vi "Z_Alignment_v12 (SubVI).vi"(4 "System no.":i32, 5 "Z range":dbl, 6 "Intensity Graph":dbl[][](array[numeric]), 7 "Z Mesh":dbl, 8 "error in (no error)":errorcluster, 9 "Z":dbl, 10 "Y":dbl, 11 "X":dbl) -> (0 "error out":errorcluster, 1 "Zout":dbl)   [LabVIEW 2023]
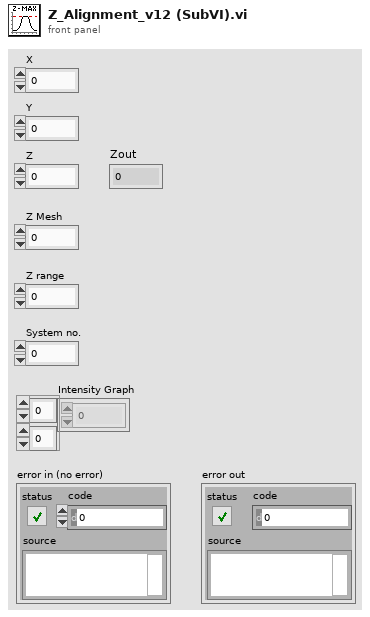
[diagram p1: front panel]
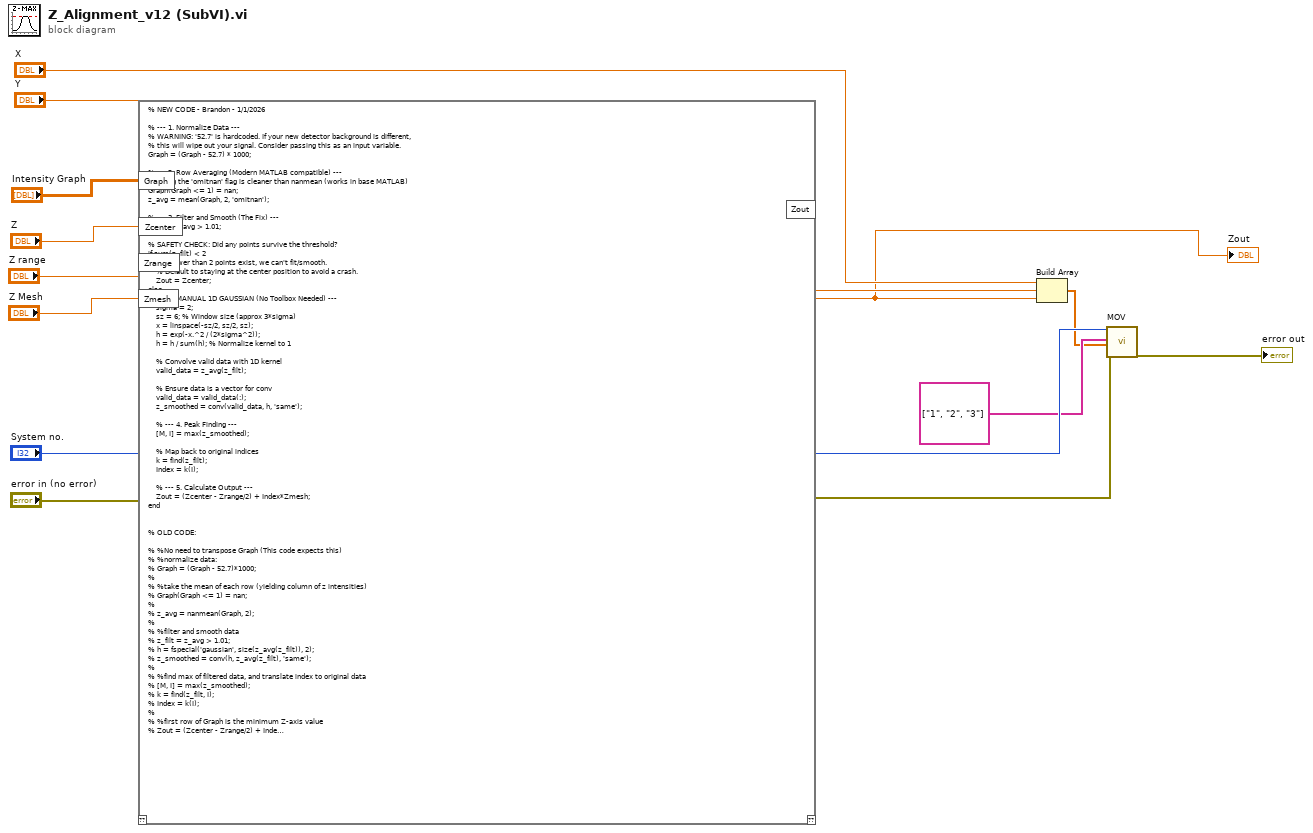
[diagram p0: block diagram]
diagram:
  n1 = script code="% NEW CODE - Brandon - 1/1/2026\n\n% --- 1. Normalize Data ---\n% WARNING: '52.7' is hardcoded. If your new detector background is different,\n% this will wipe out your signal. Consider passing this as an input variable.\nGraph = (Graph - 52.7) * 1000;\n\n% --- 2. Row Averaging (Modern MATLAB compatible) ---\n% Using the 'omitnan' flag is cleaner than nanmean (works in base MATLAB)\nGraph(Graph <= 1) = nan;\nz_avg = mean(Graph, 2, 'omitnan');\n\n% --- 3. Filter and Smooth (The Fix) ---\nz_filt = z_avg > 1.01;\n\n% SAFETY CHECK: Did any points survive the threshold?\nif sum(z_filt) < 2\n    % If fewer than 2 points exist, we can't fit/smooth. \n    % Default to staying at the center position to avoid a crash.\n    Zout = Zcenter; \nelse\n    % --- MANUAL 1D GAUSSIAN (No Toolbox Needed) ---\n    sigma = 2; \n    sz = 6; % Window size (approx 3*sigma)\n    x = linspace(-sz/2, sz/2, sz);\n    h = exp(-x.^2 / (2*sigma^2));\n    h = h / sum(h); % Normalize kernel to 1\n\n    % Convolve valid data with 1D kernel\n    valid_data = z_avg(z_filt);\n    \n    % Ensure data is a vector for conv\n    valid_data = valid_data(:); \n    z_smoothed = conv(valid_data, h, 'same');\n\n    % --- 4. Peak Finding ---\n    [M, I] = max(z_smoothed);\n    \n    % Map back to original indices\n    k = find(z_filt);\n    Index = k(I);\n\n    % --- 5. Calculate Output ---\n    Zout = (Zcenter - Zrange/2) + Index*Zmesh;\nend\n\n\n% OLD CODE:\n\n% %No need to transpose Graph (This code expects this)\n% %normalize data:\n% Graph = (Graph - 52.7)*1000;\n% \n% %take the mean of each row (yielding column of z intensities)\n% Graph(Graph <= 1) = nan;\n% \n% z_avg = nanmean(Graph, 2);\n% \n% %filter and smooth data\n% z_filt = z_avg > 1.01;\n% h = fspecial('gaussian', size(z_avg(z_filt)), 2);\n% z_smoothed = conv(h, z_avg(z_filt), 'same');\n% \n% %find max of filtered data, and translate index to original data\n% [M, I] = max(z_smoothed);\n% k = find(z_filt, I);\n% Index = k(I);\n% \n% %first row of Graph is the minimum Z-axis value\n% Zout = (Zcenter - Zrange/2) + Index*Zmesh;"("??"="error in (no error)", "Graph"="Intensity Graph", "Zcenter"="Z", "Zrange"="Z range", "Zmesh"="Z Mesh") -> ("??"=w2:errorcluster, "Zout"=w1:dbl)
  "Zout" <- w1
  n2 = Build Array("X", "Y", w1) -> (w8:dbl[])
  n3 = call "MOV.vi"("System no."="System no.", "Axes to move"=string[] ["1", "2", "3"], "Position values"=w8, "error in"=w2) -> ("error out"=→"error out":errorcluster)  [unwired: 1 in, 14 out]
